vi "write kalman history to file.vi"(8 "error in (no error)":errorcluster, 10 "kalmanQueue for output":refnum<queue>, 11 "refnum":refnum<file>) -> (0 "error out":errorcluster, 3 "refnum out":refnum<file>)   [LabVIEW 2010]
uses:
  kalman_result_scaled.ctl
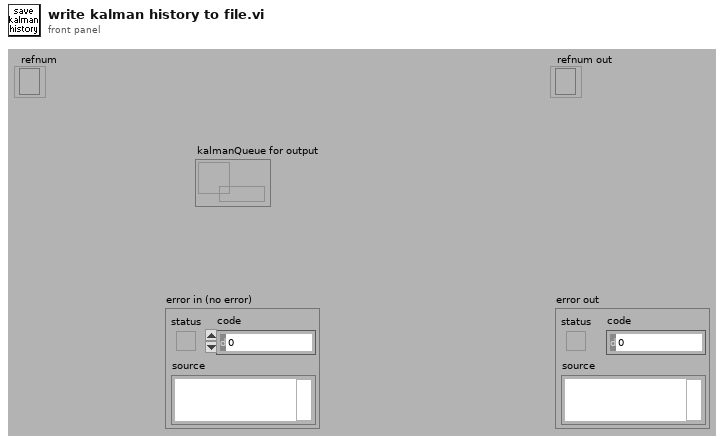
[diagram p1: front panel]
types:
  T1 = typedef "kalman_result_scaled.ctl" = cluster{"axis":u8, "pos":dbl, "vel":dbl, "wpe or z_piezo":dbl, "status":u32, "n photon ch 0":u32, "n photon ch 1":u32, "elapsed time":dbl}
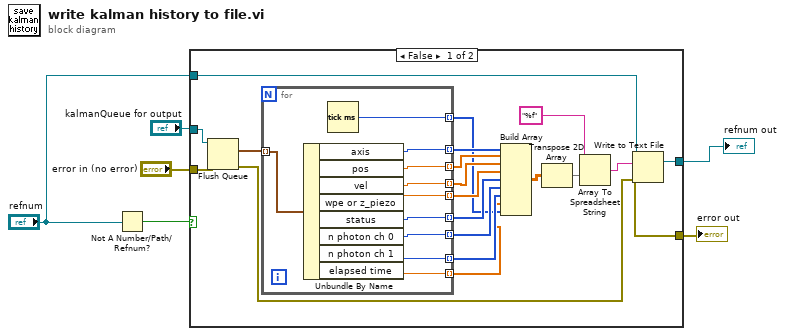
[diagram p0: block diagram]
diagram:
  n1 = Not A Number/Path/Refnum?(number/path/refnum="refnum") -> (NaN/Path/Refnum?=w3:bool)
  n2 = case shown="False" w3 {
    tunnel: "kalmanQueue for output" -> [w18 _]
    tunnel: "refnum" -> [w10 w37]
    tunnel: "error in (no error)" -> [w13 w38]
    tunnel: [w12 w38] -> w5
    tunnel: [w9 w37] -> w2
    frame False {
      n3 = Flush Queue(queue=w18, error in (no error)=w13) -> (remaining elements=w17:T1[], error out=w14:errorcluster)  [unwired: 1 out]
      n4 = for {
        tunnel: w17 -> [w36] mode=indexing
        tunnel: [w35] -> w26 mode=indexing
        tunnel: [w34] -> w25 mode=indexing
        tunnel: [w33] -> w24 mode=indexing
        tunnel: [w32] -> w23 mode=indexing
        tunnel: [w31] -> w22 mode=indexing
        tunnel: [w30] -> w21 mode=indexing
        tunnel: [w29] -> w20 mode=indexing
        tunnel: [w28] -> w19 mode=indexing
        tunnel: [w27] -> w7 mode=indexing
        n5 = Unbundle By Name(w36) -> ("axis"=w35:u8, "pos"=w34:dbl, "vel"=w33:dbl, "wpe or z_piezo"=w32:dbl, "status"=w31:u32, "n photon ch 0"=w30:u32, "n photon ch 1"=w29:u32, "elapsed time"=w28:dbl)
        n6 = Tick Count (ms)() -> (millisecond timer value=w27:u32)
      }
      n7 = Build Array(w26, w25, w24, w23, w22, w21, w20, w19, w7) -> (w16:dbl[][])
      n8 = Transpose 2D Array(2D array=w16) -> (transposed array=w8:dbl[][])
      n9 = Array To Spreadsheet String(array=w8, 3:"%f" ("format (%.3f)")) -> (spreadsheet string=w11:string)  [unwired: 1 in]
      n10 = Write to Text File(file (use dialog)=w10, text=w11, error in=w14) -> (refnum out=w9:refnum<file>, error out=w12:errorcluster)  [unwired: 1 in, 1 out]
    }
    frame True {
    }
  }
  "error out" <- w5
  "refnum out" <- w2
